vi "SR830 query sin out voltage.vi"(8 "error in (no error)":errorcluster, 11 "VISA resource name":refnum<visa-resource-name>) -> (0 "error out":errorcluster, 2 "voltage":dbl[unit], 3 "VISA resource name out":refnum<visa-resource-name>)   [LabVIEW 2009, in "SR830.lvlib"]
doc: "Reads the current voltage of the SINE OUT output of the lock-in amplifier."
uses:
  SR830.lvlib
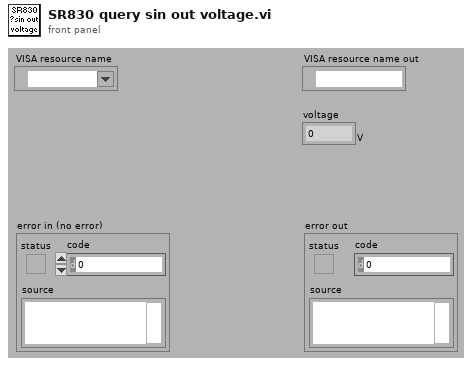
[diagram p1: front panel]
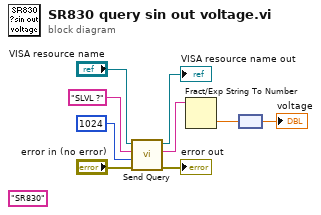
[diagram p0: block diagram]
diagram:
  (unwired) "SR830" ("name (unnamed)")
  n1 = call "Send Query.vi"("error in (no error)"="error in (no error)", "Bytes Count"=u32 1024 ("bytes to read (1000)"), "write buffer"="SLVL ?", "VISA resource name"="VISA resource name") -> ("error out"=→"error out":errorcluster, "read buffer"=w3:string, "VISA resource name out"=→"VISA resource name out":refnum<visa-resource-name>)  [unwired: 5 in]
  n2 = Fract/Exp String To Number(string=w3) -> (number=w9:dbl)  [unwired: 4 out]
  n3 = node(w9) -> (→"voltage":dbl[unit])
